vi "control lab hamdy.vi"() -> ()   [LabVIEW 2018]
uses:
  <vilib>/LabVIEW Interface for Arduino/Type Defs/Board Type.ctl
  <vilib>/LabVIEW Interface for Arduino/Type Defs/Connection Type.ctl
  <vilib>/LabVIEW Interface for Arduino/LabVIEW Interface for Arduino.lvlib
panel:
  in  "stop":bool
  out "Tank":dbl(slide) scale=0.0..100.0
  in  "Boolean":bool
  in  "VISA resource":refnum<visa-resource-name>
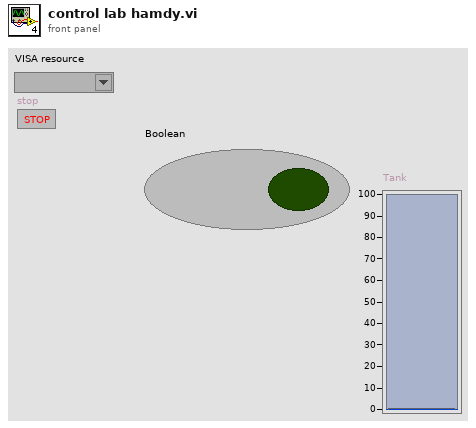
[diagram p1: front panel]
types:
  T1 = typedef "LabVIEW Interface for Arduino.lvlib/Connection Type.ctl" = enum8{"USB / Serial", "XBEE", "BlueSmirf (Bluetooth)"}
  T2 = typedef "LabVIEW Interface for Arduino.lvlib/Board Type.ctl" = enum16{"Uno", "Dimuelanove w/Atmega 328", "Mega 2560"}
  T3 = typedef "LabVIEW Interface for Arduino.lvlib/Arduino Resource.ctl" = cluster{"VISA resource":refnum<visa-resource-name>, "Board Type":T2, "Connection Type":enum8{"USB / Serial"}, "Bytes Per Packet (15)":u8}
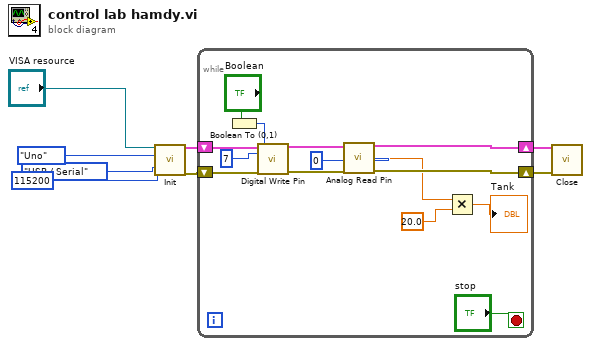
[diagram p0: block diagram]
diagram:
  n1 = call <vilib>:"Init.vi"("VISA resource"="VISA resource", "Baud Rate (115200)"=u32 115200, "Board Type (Uno)"=Board_Type."Uno", "Connection Type (USB/Serial)"=Connection_Type."USB / Serial") -> ("Arduino Resource"=w4:T3, "error out"=w3:errorcluster)  [unwired: 14 in]
  n2 = while {
    shift-right: [w14] -> w1
    shift-left: w4 -> [w22]
    shift-right: [w15] -> w2
    shift-left: w3 -> [w21]
    stop <- "stop" stop-if-true
    n3 = Boolean To (0,1)(Boolean="Boolean") -> (0, 1=w18:i16)
    n4 = call <vilib>:"Digital Write Pin.vi"("Arduino Resource"=w22, "Digital I/O Pin (0)"=u8 7, "Value (0)"=w18, "error in"=w21) -> ("Arduino Resource"=w17:T3, "error out"=w16:errorcluster)  [unwired: 10 in]
    n5 = call <vilib>:"Analog Read Pin.vi"("Arduino Resource"=w17, "Analog Input Pin (0)"=u8 0, "error in"=w16) -> ("Arduino Resource"=w14:T3, "Voltage"=w12:dbl, "error out"=w15:errorcluster)  [unwired: 10 in]
    n6 = Multiply(x=w12, y=20.0) -> (x*y=→"Tank":dbl)
  }
  n7 = call <vilib>:"Close.vi"("Arduino Resource"=w1, "error in"=w2) -> ()  [unwired: 13 in, 1 out]
